vi "reset_stage_simpler (SubVI).vi"(8 "error in (no error)":errorcluster, 11 "IP address":string) -> (0 "error out":errorcluster, 2 "deviceKey":string, 3 "reference":refnum<k24>)   [LabVIEW 2016]
uses:
  C:/Users/UsphereLab/Documents/GitHub/Optlev/LabView Code/Examples/Tilt Stage/CmdLib.dll
  Examples/Tilt Stage/CmdLib.dll
panel:
  out "Numeric":i32
  out "deviceKeys":string[](array[string])
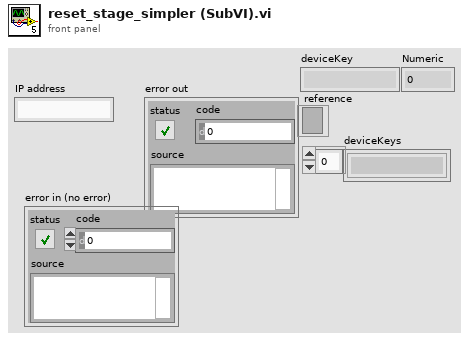
[diagram p1: front panel]
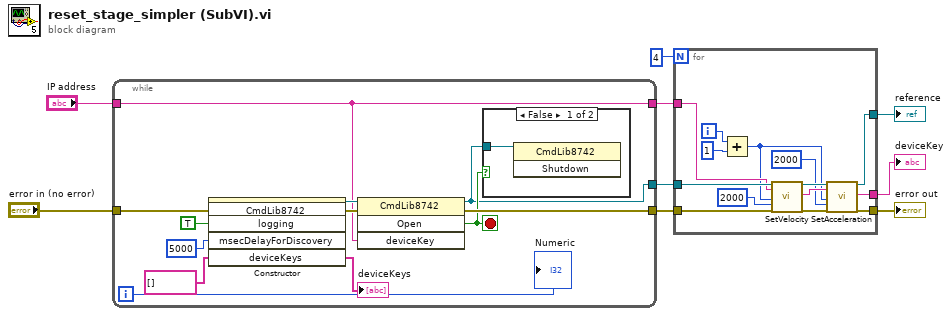
[diagram p0: block diagram]
diagram:
  n1 = while {
    tunnel: [w17] -> w6
    tunnel: "IP address" -> [w14]
    tunnel: [w14] -> w5
    tunnel: [w15] -> w7
    tunnel: "error in (no error)" -> [w11]
    i -> [w10]
    stop <- w16 stop-if-true
    n2 = constructor class="CmdLib8742"(error in=w11, "logging"=TRUE, "msecDelayForDiscovery"=5000, "deviceKeys"=string[] []) -> (reference out=w19:refnum<k24>, error out=w18:errorcluster, "deviceKeys"=→"deviceKeys":string[])  [unwired: 2 in, 3 out]
    n3 = invoke class="CmdLib8742" method="Open"(reference=w19, error in=w18, "deviceKey"=w14) -> (reference out=w15:refnum<k24>, error out=w17:errorcluster, "Open"=w16:bool)  [unwired: 1 in, 1 out]
    n4 = case shown="False" w16 {
      tunnel: w15 -> [w22 _]
      frame False {
        n5 = invoke class="CmdLib8742" method="Shutdown"(reference=w22) -> ()  [unwired: 2 in, 3 out]
      }
      frame True {
      }
    }
    "Numeric" <- w10
  }
  n6 = for {
    N: 4 -> [_]
    tunnel: w7 -> [w36]
    tunnel: w6 -> [w35]
    tunnel: w5 -> [w34]
    tunnel: [w25] -> w4
    tunnel: [w24] -> w3
    tunnel: [w23] -> w2
    i -> [w33]
    n7 = Add(x=w33, y=1) -> (x+y=w28:i32)
    n8 = call "SetVelocity.vi"("CmdLib In"=w36, "DeviceKey In"=w34, "Motor"=w28, "Steps Per Sec"=2000, "error in (no error)"=w35) -> ("CmdLib Out"=w30:refnum<k24>, "DeviceKey Out"=w29:string, "error out"=w26:errorcluster)  [unwired: 11 in, 1 out]
    n9 = call "SetAcceleration.vi"("CmdLib In"=w30, "DeviceKey In"=w29, "Motor"=w28, "Steps Per Sec 2"=2000, "error in (no error)"=w26) -> ("CmdLib Out"=w24:refnum<k24>, "DeviceKey Out"=w23:string, "error out"=w25:errorcluster)  [unwired: 11 in, 1 out]
  }
  "error out" <- w4
  "deviceKey" <- w2
  "reference" <- w3
